vi "PAUSE.vi"(0 "VISA resource name":refnum<visa-resource-name>, 5 "Pause Time (s)":string, 7 "Command Terminator":bool=TRUE, 11 "error in (no error)":errorcluster) -> (4 "VISA resource name out":refnum<visa-resource-name>, 6 "Command Output":string, 8 "Error Message":string, 10 "Error Code":i32, 15 "error out":errorcluster)   [LabVIEW 2010, in "VITREK V7X.lvlib"]
doc: "Configures the <b>PAUSE</b> input.\n\n<b>Note:</b> please refer to the instrument manual for the <b>PASUE</b> input specification."
uses:
  VITREK V7X.lvlib
panel:
  # "Yes\n\nNo"
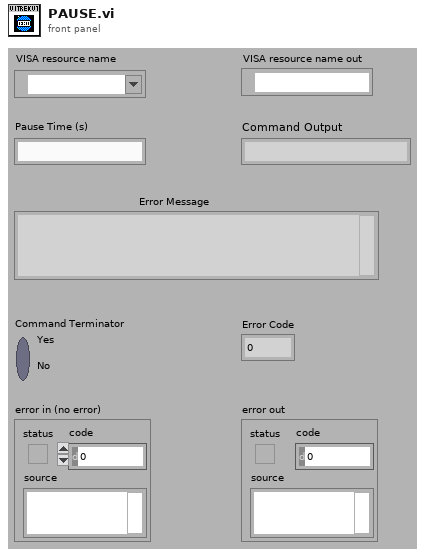
[diagram p1: front panel]
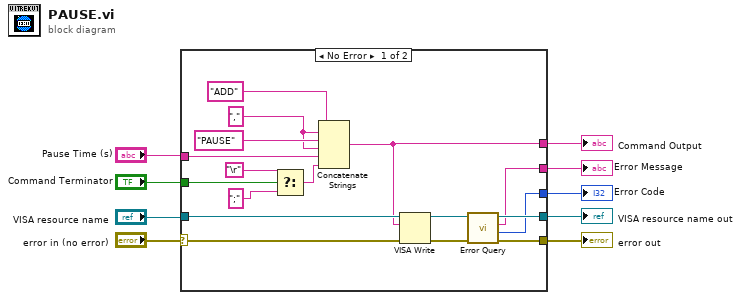
[diagram p0: block diagram]
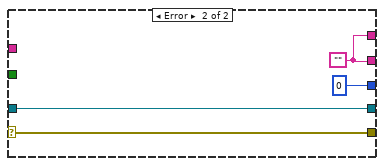
[diagram p2: hidden frame]
diagram:
  n1 = case shown="No Error" "error in (no error)" {
    selector: "error in (no error)" -> [w21 w29]
    tunnel: "VISA resource name" -> [w26 w30]
    tunnel: [w19 w27] -> w8
    tunnel: [w23 w30] -> w7
    tunnel: [w22 w29] -> w6
    tunnel: "Pause Time (s)" -> [w13 _]
    tunnel: "Command Terminator" -> [w18 _]
    tunnel: [w11 0 ("Error Code")] -> w2
    tunnel: [w10 w27] -> w1
    frame No Error {
      w14 = ","
      n2 = Select(t="\r", s=w18, f=";") -> (s? t:f=w12:string)
      n3 = Concatenate Strings("ADD", w14, "PAUSE", w14, w13, w12) -> (w19:string)
      n4 = VISA Write(VISA resource name=w26, write buffer=w19, error in (no error)=w21) -> (VISA resource name out=w25:refnum<visa-resource-name>, error out=w24:errorcluster)  [unwired: 1 out]
      n5 = call "Error Query.vi"("error in (no error)"=w24, "VISA resource name"=w25) -> ("error out"=w22:errorcluster, "Error Code"=w11:i32, "Error Message"=w10:string, "VISA resource name out"=w23:refnum<visa-resource-name>)  [unwired: 6 in]
    }
    frame Error {
      w27 = ""
    }
  }
  "VISA resource name out" <- w7
  "error out" <- w6
  "Command Output" <- w8
  "Error Code" <- w2
  "Error Message" <- w1
